vi "Requests.vi"(8 "error in (no error)":errorcluster, 9 "write enable":bool=TRUE, 11 "ICPCON ET7042 in":refnum<class "ICPCON ET-7042.lvclass">) -> (0 "error out":errorcluster, 3 "ICPCON ET7042 out":refnum<class "ICPCON ET-7042.lvclass">)   [LabVIEW 2021, in "ICPCON ET-7042.lvclass"]
uses:
  ICPCON ET-7042.lvclass
  D:/my_projects/projects/Algorithms/Labview/21/Modbus_v121c/Network Protocol/MB/Modbus Master CR.lvclass
  D:/my_projects/projects/Algorithms/Labview/21/Modbus_v121c/Network Protocol/Network Master/Network Master.lvclass
  MB/Modbus Master CR.lvclass/Modbus Master CR.ctl
  Modbus Data Unit/Modbus Data Unit.lvclass/Modbus Data Unit.ctl
  Network Master/Network Master.lvclass/Network Master.ctl
  Master Function Definition/Read Coils Request.vi
  Network Master/Read write Master.vi
  Master Function Definition/Read Coils Response.vi
  Master Function Definition/Write Multiple Coils Request.vi
  Master Function Definition/Function data mismatch error.vi
  Master Function Definition/Write Multiple Coils Response.vi
  Modbus Data Unit/Construct PDU.vi
  Utility/Bytes to Bits.vi
  Data Model/Error Generator.vi
  Master Function Definition/Function code mismatch error.vi
  Modbus Data Unit/Deconstruct PDU.vi
  Utility/Bits to Bytes.vi
  Modbus Data Unit/Modbus Data Unit.lvclass
  Data Model/Device Data Model.lvclass
  Transmission Data Unit/Transmission Data Unit.lvclass
  MB/Modbus Master CR.lvclass
  Network Master/Network Master.lvclass
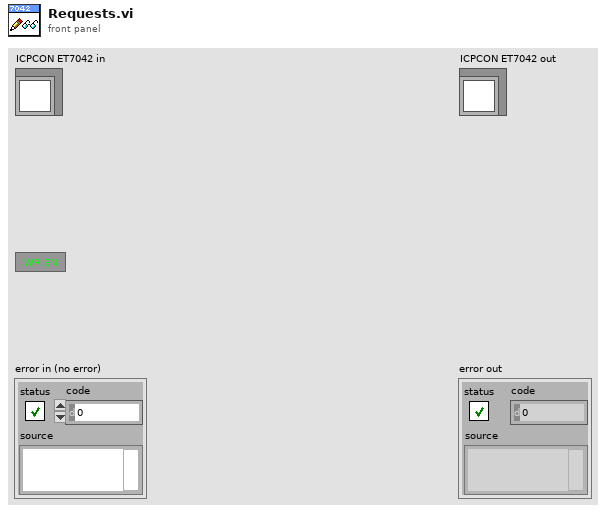
[diagram p1: front panel]
types:
  T1 = typedef "Modbus Master CR.lvclass/N channel.ctl" = cluster{"N DI channel":u16, "N DO channel":u16, "N AI channel":u16, "N AO channel":u16}
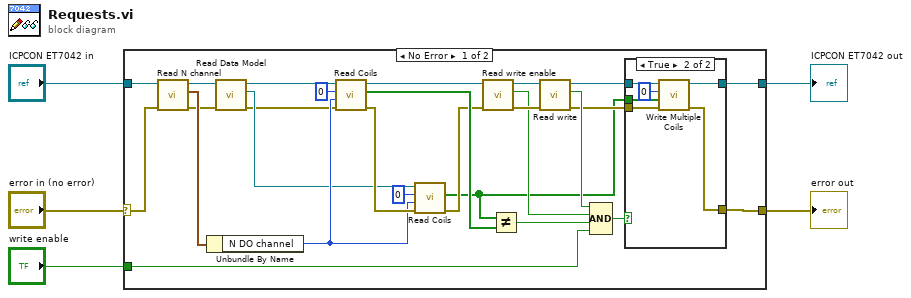
[diagram p0: block diagram]
diagram:
  n1 = case shown="No Error" "error in (no error)" {
    selector: "error in (no error)" -> [w29 w42]
    tunnel: [w15 w42] -> w3
    tunnel: [w7 w41] -> w4
    tunnel: "ICPCON ET7042 in" -> [w31 w41]
    tunnel: "write enable" -> [w16 _]
    frame No Error {
      n2 = call "Read N channel.vi"("error in (no error)"=w29, "MB_v2 in"=w31) -> ("error out"=w28:errorcluster, "N channel"=w32:T1, "MB_v2 out"=w30:refnum<class "ICPCON ET-7042.lvclass">)  [unwired: 7 in]
      n3 = Unbundle By Name(w32) -> ("N DO channel"=w18:u16)
      n4 = call "Read Data Model.vi"("error in (no error)"=w28, "MB_TCP in"=w30) -> ("error out"=w10:errorcluster, "Data Model"=w14:refnum<class "Device Data Model.lvclass">, "MB_TCP out"=w11:refnum<class "ICPCON ET-7042.lvclass">)  [unwired: 7 in]
      n5 = call "Read Coils.vi"("error in (no error)"=w10, "number of coils"=w18, "starting address"=u16 0, "Modbus master in"=w11) -> ("error out"=w20:errorcluster, "coil values"=w21:bool[], "Modbus master out"=w9:refnum<class "ICPCON ET-7042.lvclass">)  [unwired: 5 in]
      n6 = call-dynamic "Read Coils.vi"("error in"=w20, "number of coils"=w18, "starting address"=u16 0, "device data model in"=w14) -> ("error out"=w13:errorcluster, "data"=w6:bool[])  [unwired: 5 in, 1 out]
      n7 = call "Read write enable.vi"("error in (no error)"=w13, "MB in"=w9) -> ("error out"=w26:errorcluster, "write enable"=w22:bool, "MB out"=w27:refnum<class "ICPCON ET-7042.lvclass">)  [unwired: 7 in]
      n8 = Not Equal?(x=w6, y=w21) -> (x != y?=w25:bool)
      n9 = call "Read write.vi"("error in (no error)"=w26, "MB in"=w27) -> ("error out"=w12:errorcluster, "Write"=w23:bool, "MB out"=w8:refnum<class "ICPCON ET-7042.lvclass">)  [unwired: 7 in]
      n10 = Compound Arithmetic op=AND(w23, w22, w25, w16) -> (w24:bool)
      n11 = case shown="True" w24 {
        tunnel: w12 -> [w34 w39]
        tunnel: [w34 w36] -> w15
        tunnel: w6 -> [_ w38]
        tunnel: w8 -> [w33 w40]
        tunnel: [w33 w35] -> w7
        frame False {
        }
        frame True {
          n12 = call "Write Multiple Coils.vi"("error in (no error)"=w39, "coil values"=w38, "starting address"=u16 0, "Modbus master in"=w40) -> ("error out"=w36:errorcluster, "Modbus master out"=w35:refnum<class "ICPCON ET-7042.lvclass">)  [unwired: 6 in]
        }
      }
    }
    frame Error {
    }
  }
  "error out" <- w3
  "ICPCON ET7042 out" <- w4
